vi "Ejercicio 1.1.vi"() -> ()   [LabVIEW 2020]
panel:
  in  "stop 4":bool
  in  "stop 3":bool
  in  "stop 2":bool
  in  "stop":bool
  out "LED 6":bool
  out "LED 5":bool
  out "LED 4":bool
  out "LED 3":bool
  out "LED 2":bool
  out "LED":bool
  in  "Boolean 6":bool
  in  "Boolean 5":bool
  in  "Boolean 4":bool
  in  "Boolean 3":bool
  in  "Boolean 2":bool
  in  "Boolean":bool
  # "Switch when pressed"
  # "Latch when preseed"
  # "Switch when released"
  # "Latch when released"
  # "Switch until released"
  # "Latch until released"
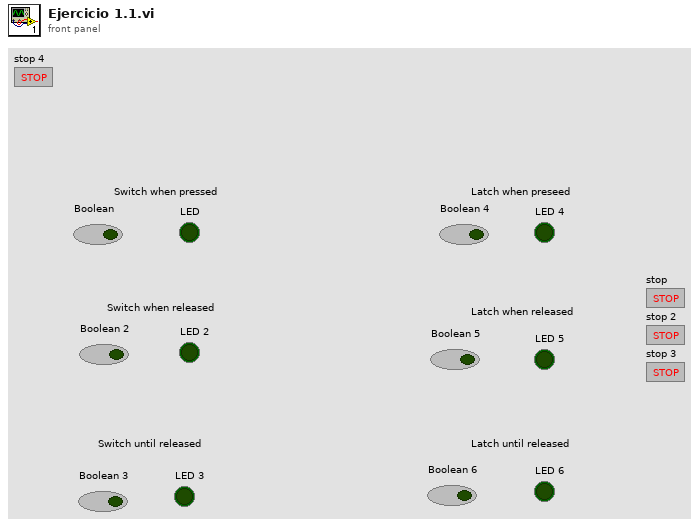
[diagram p1: front panel]
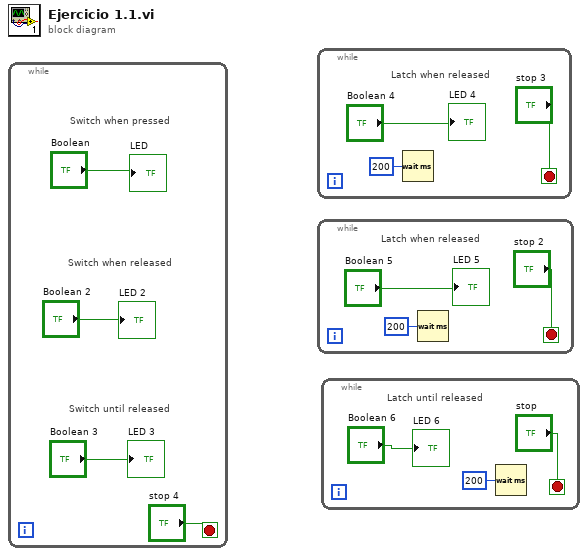
[diagram p0: block diagram]
diagram:
  n1 = while {
    stop <- "stop 4" stop-if-true
    # "Switch until released"
    # "Switch when released"
    # "Switch when pressed"
    "LED" <- "Boolean"
    "LED 2" <- "Boolean 2"
    "LED 3" <- "Boolean 3"
  }
  n2 = while {
    stop <- "stop 3" stop-if-true
    # "Latch when released"
    n3 = Wait (ms)(milliseconds to wait=u32 200) -> ()  [unwired: 1 out]
    "LED 4" <- "Boolean 4"
  }
  n4 = while {
    stop <- "stop 2" stop-if-true
    # "Latch when released"
    n5 = Wait (ms)(milliseconds to wait=u32 200) -> ()  [unwired: 1 out]
    "LED 5" <- "Boolean 5"
  }
  n6 = while {
    stop <- "stop" stop-if-true
    # "Latch until released"
    n7 = Wait (ms)(milliseconds to wait=u32 200) -> ()  [unwired: 1 out]
    "LED 6" <- "Boolean 6"
  }
